vi "2.2 Steering Chooser.vi"(10 "Waypoint":T5, 11 "Waypoint Queue In":T1) -> ()   [LabVIEW 2011]
doc: "Takes waypoint and boat location information from the global variable and places the approproate rudder position command on the global.\nFor Drive waypoints, this VI simply tries to make the boat's heading the same as the heading between the boat and the waypoint. TODO: this does not account for drift -- it assumes that the boat will go where it is pointed which is not always the case.\n\nTODO: important: As of 11/17 this VI only works for the Drive option.\nTODO: ideally this VI would run on any update of the boat location or waypoint location, and not otherwise."
uses:
  2 Typedefs/heading.ctl
  2x3-RIO-OCU Comm/2x3 Typedefs/ocuWaypoint.ctl
  2x3-RIO-OCU Comm/2x3 Typedefs/waypointTypes.ctl
  2 Typedefs/UTM Location.ctl
  2 Typedefs/Velocity.ctl
  2x3-RIO-OCU Comm/2x3 Typedefs/waypointQueue.ctl
  2 Globals/2 Global.vi
panel:
  out "Robot\nHeading":T2 format="%05.1f"
  out "Angle to waypt":T2 format="%05.1f"
  out "Distance to Waypoint":T3
  out "Robot UTM Location":T4
  out "desired delta heading":T2 format="%05.1f"
  # "Steering Chooser simply turns the rudder to aim the boat's bow towards the next waypoint.\n\nTODO: currently only implements Drive waypoints. Also this is extremely stupid.\nImplement avoidance, stay-in-area, and maybe a PID loop."
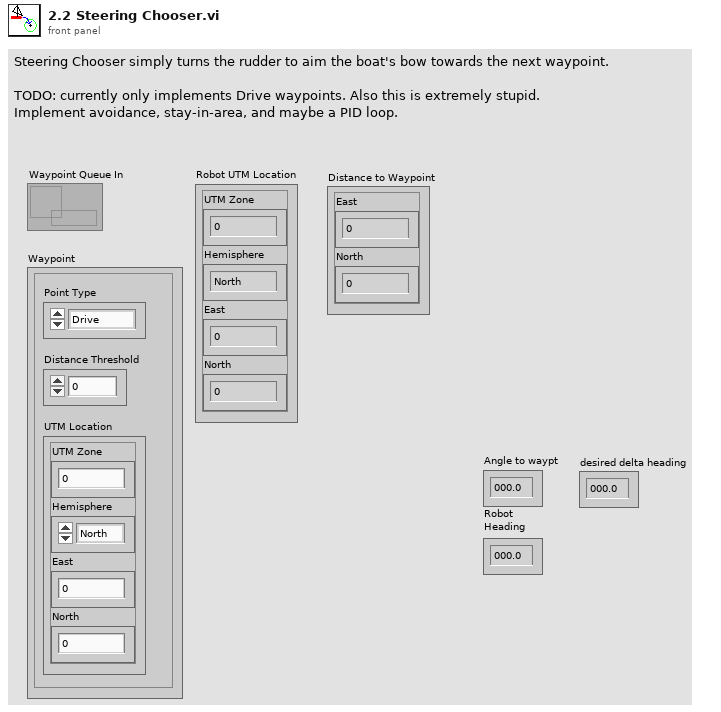
[diagram p1: front panel]
types:
  T1 = typedef "waypointQueue.ctl" = refnum<queue>
  T2 = typedef "heading.ctl" = dbl
  T3 = typedef "Velocity.ctl" = cluster{"East":dbl, "North":dbl}
  T4 = typedef "UTM Location.ctl" = cluster{"UTM Zone":dbl, "Hemisphere":enum16{"North", "South"}, "East":dbl, "North":dbl}
  T5 = typedef "ocuWaypoint.ctl" = cluster{"Point Type":T6, "Distance Threshold":dbl, "UTM Location":T4}
  T6 = typedef "waypointTypes.ctl" = enum16{"Drive", "Round Port", "Round Starboard", "Stay"}
  T7 = cluster{"UTM Zone":dbl, "Hemisphere":u16, "East":dbl, "North":dbl}
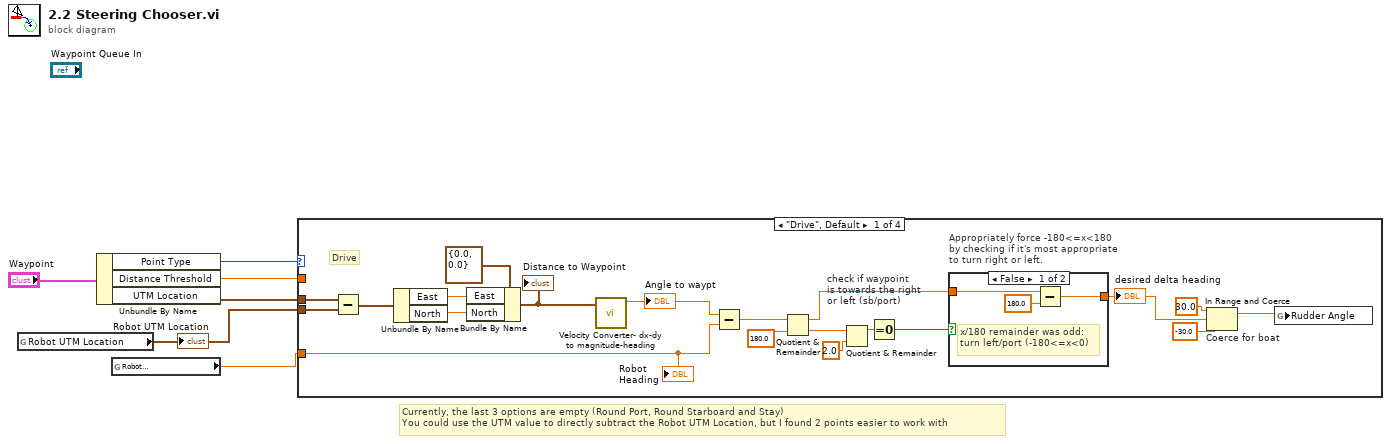
[diagram p0: block diagram]
diagram:
  # "Currently, the last 3 options are empty (Round Port, Round Starboard and Stay)\nYou could use the UTM value to directly subtract the Robot UTM Location, but I found 2 points easier to work with"
  n1 = global read "2 Global.vi" "Robot UTM Location"() -> (w6:T4)
  "Robot UTM Location" <- w6
  n2 = Unbundle By Name("Waypoint") -> ("Point Type"=w2:T6, "Distance Threshold"=w3:dbl, "UTM Location"=w4:T4)
  n3 = global read "2 Global.vi" "Robot\nHeading"() -> (w5:T2)
  n4 = case shown="\"Drive\", Default" w2 {
    tunnel: w4 -> [w26 _ _ _]
    tunnel: w6 -> [w25 _ _ _]
    tunnel: w5 -> [w19 _ _ _]
    tunnel: w3 -> [_ _ _ _]
    frame "Drive", Default {
      # "Drive"
      n5 = Subtract(x=w26, y=w25) -> (x-y=w24:T7)
      n6 = Unbundle By Name(w24) -> ("East"=w23:dbl, "North"=w22:dbl)
      n7 = Bundle By Name(cluster=T3 {"East"=0.0, "North"=0.0} ("Vector In"), "East"=w23, "North"=w22) -> (w20:T3)
      "Distance to Waypoint" <- w20
      n8 = call "Velocity Converter- dx-dy to magnitude-heading.vi"("Vector In"=w20) -> ("Heading Out"=w15:T2)  [unwired: 9 in, 1 out]
      "Angle to waypt" <- w15
      n9 = Subtract(x=w15, y=w19) -> (x-y=w13:T2)
      n10 = Quotient & Remainder ("shift to -180<x<180")(x=w13, y=T2 180.0) -> (x-y*floor(x/y)=w8:T2, floor(x/y)=w12:T2)
      n11 = Quotient & Remainder ("shift to -180<x<180")(x=w12, y=T2 2.0) -> (x-y*floor(x/y)=w10:T2)  [unwired: 1 out]
      n12 = Equal To 0? "check if waypoint\nis towards the right\nor left (sb/port)"(x=w10) -> (x = 0?=w9:bool)
      n13 = case "Appropriately force -180<=x<180\nby checking if it's most appropriate\nto turn right or left." shown="False" w9 {
        tunnel: w8 -> [w28 w30]
        tunnel: [w27 w30] -> w7
        frame False {
          # "x/180 remainder was odd:\nturn left/port (-180<=x<0)"
          n14 = Subtract(x=w28, y=T2 180.0) -> (x-y=w27:T2)
        }
        frame True {
          # "x/180 remainder was\neven: turn right/sb\n(0<=x<180)"
        }
      }
      "desired delta heading" <- w7
      n15 = In Range and Coerce "Coerce for boat"(upper limit=T2 30.0, x=w7, lower limit=T2 -30.0) -> (coerced(x)=w16:T2)  [unwired: 1 out]
      n16 = global write "2 Global.vi" "Rudder Angle"(w16) -> ()
      "Robot\nHeading" <- w19
    }
    frame "Round Port" {
      # "Round Port"
    }
    frame "Round Starboard" {
      # "Round Starboard"
    }
    frame "Stay" {
      # "Stay"
    }
  }
